vi "Int_to_Enum.vi"(11 "IntIn":i32) -> (3 "EnumOut":T1)   [LabVIEW 2015]
uses:
  AutoMode.ctl
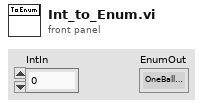
[diagram p1: front panel]
types:
  T1 = typedef "AutoMode.ctl" = enum16{"OneBallFront", "OneBallCollector", "TwoBallNormal", "TwoBallHot"}
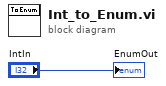
[diagram p0: block diagram]
diagram:
  "EnumOut" <- "IntIn"
